vi "Array of Register.vi"(8 "Register":i32, 9 "Registers":T3[](array[typedef]) format="%032b", 10 "Arrays":T1 {"Array" format="%032b"}) -> (2 "Array":T2 format="%032b")   [LabVIEW 2020]
uses:
  Platter.ctl
  Array.ctl
  Arrays.ctl
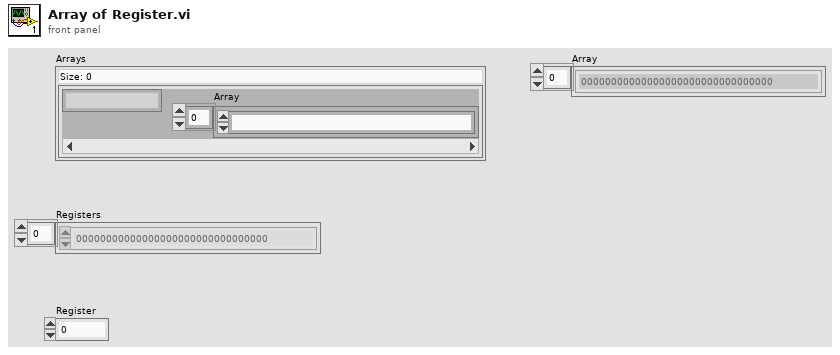
[diagram p1: front panel]
types:
  T1 = typedef "Arrays.ctl" = map{string, T2}
  T2 = typedef "Array.ctl" = T3[]
  T3 = typedef "Platter.ctl" = u32
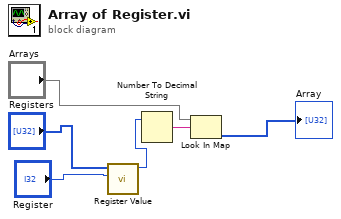
[diagram p0: block diagram]
diagram:
  n1 = call "Register Value.vi"("Register"="Register", "Registers"="Registers") -> ("Platter"=w1:T3)  [unwired: 9 in]
  n2 = Number To Decimal String(number=w1) -> (decimal integer string=w5:string)  [unwired: 1 in]
  n3 = Look In Map(map="Arrays", key=w5) -> (value=→"Array":T2)  [unwired: 1 in, 1 out]
